vi "onTestExecution.vi"(6 "timeout (2000 ms)":i32=2000, 7 "Name":string, 8 "error in (no error)":errorcluster, 11 "DMC Folder Test Runner in":refnum<class "DMC Folder Test Runner.lvclass">) -> (0 "error out":errorcluster, 3 "DMC Folder Test Runner out":refnum<class "DMC Folder Test Runner.lvclass">)   [LabVIEW 2023, in "DMC Folder Test Runner.lvclass"]
uses:
  DMC Folder Test Runner.lvclass
  <vilib>/addons/_JKI Toolkits/Caraya/classes/Test Runner/Test Runner.lvclass/Test Runner.ctl
  <vilib>/addons/_JKI Toolkits/Caraya/classes/Assert/Assert Not Error.vi
  DMC Folder Test Runner.lvclass/DMC Folder Test Runner.ctl
  <vilib>/addons/_JKI Toolkits/Caraya/classes/Test/Test.lvclass
  <vilib>/addons/_JKI Toolkits/Caraya/classes/Assert/Assert.lvclass
  <vilib>/addons/_JKI Toolkits/Caraya/classes/Test Runner/Test Runner.lvclass
  C:/Program Files/National Instruments/LabVIEW 2023/vi.lib/addons/_JKI Toolkits/Caraya/classes/Test Runner.Folder/Test Runner.Folder.lvclass
  C:/Program Files/National Instruments/LabVIEW 2023/vi.lib/addons/_JKI Toolkits/Caraya/classes/Test Runner/Test Runner.lvclass
  C:/Projects/Open Source/DMC CLI - Caraya/Source/DMC Folder Test Runner/DMC Folder Test Runner.lvclass
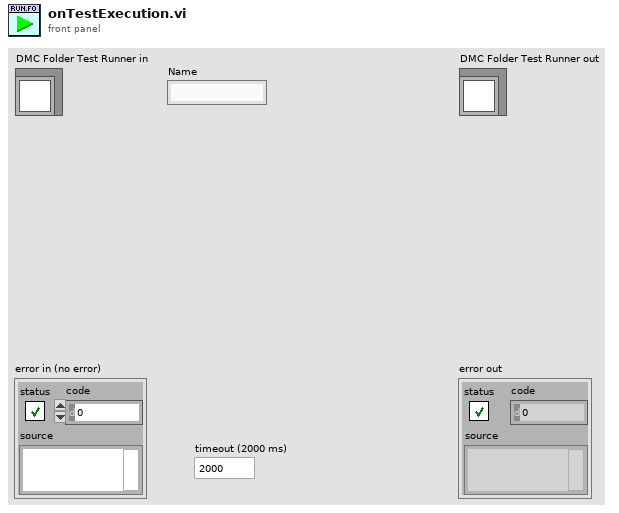
[diagram p1: front panel]
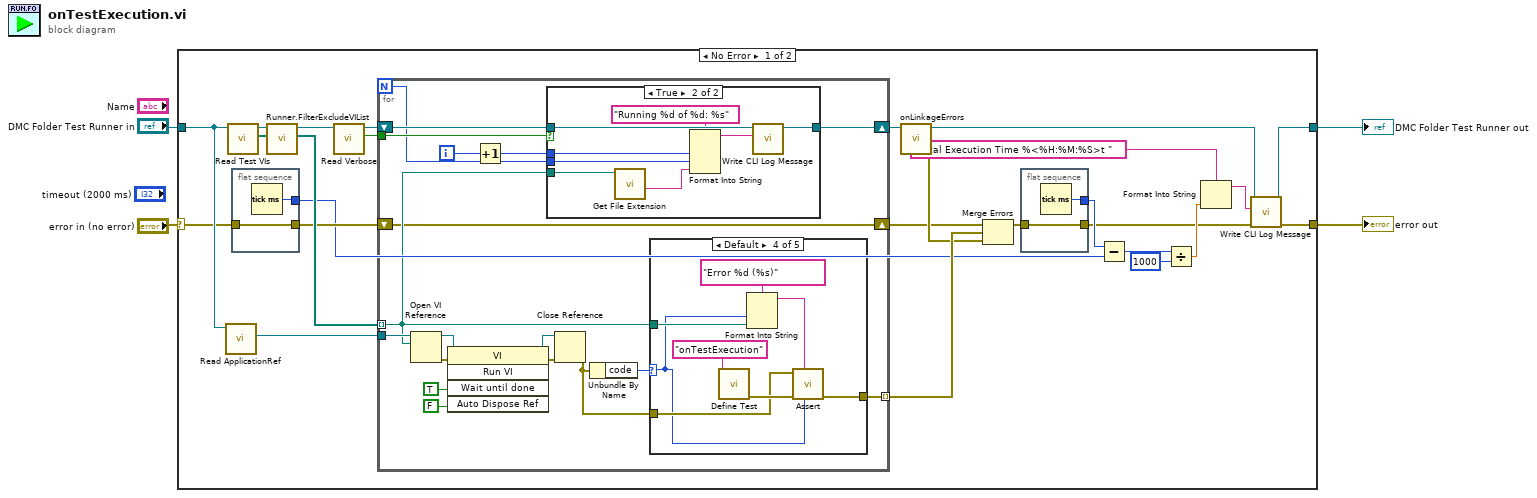
[diagram p0: block diagram]
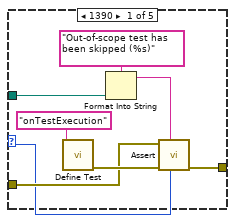
[diagram p3: hidden frame]
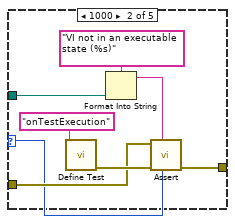
[diagram p4: hidden frame]
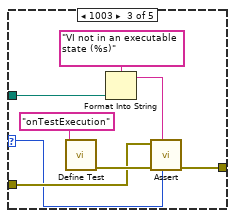
[diagram p5: hidden frame]
diagram:
  n1 = case shown="No Error" "error in (no error)" {
    selector: "error in (no error)" -> [w19 w96]
    tunnel: "DMC Folder Test Runner in" -> [w25 w95]
    tunnel: [w8 w95] -> w3
    tunnel: [w7 w96] -> w4
    frame No Error {
      n2 = call <vilib>:"Read ApplicationRef.vi"("Test Runner in"=w25) -> ("Application"=w29:refnum<vi>)  [unwired: 8 in, 2 out]
      n3 = call <vilib>:"Read Test VIs.vi"("Test Runner in"=w25) -> ("Test VIs"=w27:path[], "Test Runner out"=w24:refnum<class "DMC Folder Test Runner.lvclass">)  [unwired: 8 in, 1 out]
      n4 = flat-sequence {
        tunnel: [w34] -> w18
        tunnel: w19 -> [w34]
        tunnel: [w33] -> w11
        frame #0 {
          n5 = Tick Count (ms)() -> (millisecond timer value=w33:u32)
        }
      }
      n6 = call <vilib>:"Runner.FilterExcludeVIList.vi"("Paths"=w27, "Test Runner"=w24) -> ("Filtered Paths"=w26:path[], "Test Runner"=w22:refnum<class "DMC Folder Test Runner.lvclass">)  [unwired: 8 in]
      n7 = call <vilib>:"Read Verbose.vi"("Test Runner in"=w22) -> ("Verbose"=w20:bool, "Test Runner out"=w21:refnum<class "DMC Folder Test Runner.lvclass">)  [unwired: 9 in]
      n8 = for {
        N -> [w39]
        tunnel: w26 -> [w36] mode=indexing
        tunnel: [w52] -> w30 mode=indexing
        tunnel: w29 -> [w51]
        shift-right: [w41] -> w23
        shift-left: w21 -> [w42]
        tunnel: w20 -> [w40]
        shift-right: [w35] -> w17
        shift-left: w18 -> [w35]
        i -> [w38]
        n9 = Open VI Reference(application reference (local)=w51, vi path=w36) -> (vi reference=w43:refnum<vi>, error out=w50:errorcluster)  [unwired: 4 in]
        n10 = invoke on="Invoke Node" class="VI" method="Run VI"(reference=w43, error in=w50, "Wait until done"=TRUE ("Wait Until Done"), "Auto Dispose Ref"=FALSE ("Auto Dispose Reference")) -> (reference out=w46:refnum<vi>, error out=w45:errorcluster)  [unwired: 1 in, 3 out]
        n11 = Increment(x=w38) -> (x+1=w37:i32)
        n12 = case shown="True" w40 {
          tunnel: w42 -> [w53 w61]
          tunnel: [w53 w60] -> w41
          tunnel: w39 -> [_ w56]
          tunnel: w37 -> [_ w55]
          tunnel: w36 -> [_ w54]
          frame False {
          }
          frame True {
            n13 = call <vilib>:"Get File Extension.vi"("file"=w54) -> ("filename without extension"=w58:string)  [unwired: 6 in, 4 out]
            n14 = Format Into String(format string="Running %d of %d: %s", w55, w56, w58) -> (resulting string=w57:string)  [unwired: 2 in, 1 out]
            n15 = call "Write CLI Log Message.vi"("Message"=w57, "DMC Folder Test Runner in"=w61) -> ("DMC Folder Test Runner out"=w60:refnum<class "DMC Folder Test Runner.lvclass">)  [unwired: 8 in, 1 out]
          }
        }
        n16 = Close Reference(reference=w46, error in (no error)=w45) -> (error out=w44:errorcluster)
        n17 = Unbundle By Name(w44) -> ("code"=w47:i32)
        n18 = case shown="Default" w47 {
          selector: w47 -> [w62 w70 w78 w86 _]
          tunnel: w44 -> [w63 w71 w79 w87 w94]
          tunnel: [w65 w73 w81 w90 w94] -> w52
          tunnel: w36 -> [w69 w77 w85 w93 _]
          frame 1390 {
            n19 = call <vilib>:"Define Test.vi"("Label (VI Title)"="onTestExecution" ("Label")) -> ("error out"=w66:errorcluster)  [unwired: 9 in, 1 out]
            n20 = Format Into String(format string="Out-of-scope test has been skipped (%s)" ("Label"), w69) -> (resulting string=w64:string)  [unwired: 2 in, 1 out]
            n21 = call-poly <vilib>:"Assert.vi"("error code (1)"=w62, "Label"=w64, "error in (no error)"=w66, "Not Error?"=w63) -> ("error out"=w65:errorcluster)  [unwired: 6 in, 1 out]
          }
          frame 1000 {
            n22 = call <vilib>:"Define Test.vi"("Label (VI Title)"="onTestExecution" ("Label")) -> ("error out"=w74:errorcluster)  [unwired: 9 in, 1 out]
            n23 = Format Into String(format string="VI not in an executable state (%s)" ("Label"), w77) -> (resulting string=w72:string)  [unwired: 2 in, 1 out]
            n24 = call-poly <vilib>:"Assert.vi"("error code (1)"=w70, "Label"=w72, "error in (no error)"=w74, "Not Error?"=w71) -> ("error out"=w73:errorcluster)  [unwired: 6 in, 1 out]
          }
          frame 1003 {
            n25 = call <vilib>:"Define Test.vi"("Label (VI Title)"="onTestExecution" ("Label")) -> ("error out"=w82:errorcluster)  [unwired: 9 in, 1 out]
            n26 = Format Into String(format string="VI not in an executable state (%s)" ("Label"), w85) -> (resulting string=w80:string)  [unwired: 2 in, 1 out]
            n27 = call-poly <vilib>:"Assert.vi"("error code (1)"=w78, "Label"=w80, "error in (no error)"=w82, "Not Error?"=w79) -> ("error out"=w81:errorcluster)  [unwired: 6 in, 1 out]
          }
          frame Default {
            n28 = call <vilib>:"Define Test.vi"("Label (VI Title)"="onTestExecution" ("Label")) -> ("error out"=w88:errorcluster)  [unwired: 9 in, 1 out]
            n29 = Format Into String(format string="Error %d (%s)" ("Label"), w86, w93) -> (resulting string=w89:string)  [unwired: 2 in, 1 out]
            n30 = call-poly <vilib>:"Assert.vi"("error code (1)"=w86, "Label"=w89, "error in (no error)"=w88, "Not Error?"=w87) -> ("error out"=w90:errorcluster)  [unwired: 6 in, 1 out]
          }
          frame 0 {
          }
        }
      }
      n31 = call-dynamic "onLinkageErrors.vi"("Test Runner in"=w23) -> ("error out"=w28:errorcluster, "Test Runner out"=w9:refnum<class "DMC Folder Test Runner.lvclass">)  [unwired: 9 in]
      n32 = Merge Errors(w17, w30, w28) -> (w16:errorcluster)
      n33 = flat-sequence {
        tunnel: [w32] -> w6
        tunnel: w16 -> [w32]
        tunnel: [w31] -> w12
        frame #0 {
          n34 = Tick Count (ms)() -> (millisecond timer value=w31:u32)
        }
      }
      n35 = Subtract(x=w12, y=w11) -> (x-y=w13:u32)
      n36 = Divide(x=w13, y=u32 1000) -> (x/y=w10:dbl)
      n37 = Format Into String(format string="Total Execution Time %<%H:%M:%S>t ", w10) -> (resulting string=w5:string)  [unwired: 2 in, 1 out]
      n38 = call "Write CLI Log Message.vi"("error in (no error)"=w6, "Message"=w5, "DMC Folder Test Runner in"=w9) -> ("error out"=w7:errorcluster, "DMC Folder Test Runner out"=w8:refnum<class "DMC Folder Test Runner.lvclass">)  [unwired: 7 in]
    }
    frame Error {
    }
  }
  "error out" <- w4
  "DMC Folder Test Runner out" <- w3
